vi "AddVI.vi"() -> ()   [LabVIEW 2023]
panel:
  out "Sum":dbl
  in  "B":dbl
  in  "A":dbl
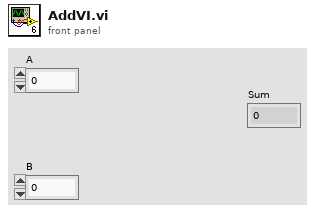
[diagram p1: front panel]
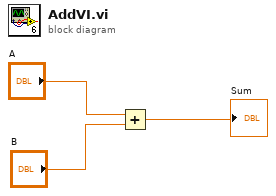
[diagram p0: block diagram]
diagram:
  n1 = Add(x="A", y="B") -> (x+y=→"Sum":dbl)
